vi "stop.vi"(3 "error in (no error)":errorcluster, 4 "stop":bool, 5 "niDAQmxAO in":refnum<class "niDAQmxAO.lvclass">) -> (0 "error out":errorcluster, 1 "Stopped":bool, 2 "niDAQmxAO out":refnum<class "niDAQmxAO.lvclass">)   [LabVIEW 2009, in "Hardware.lvlib" / "Channels.lvlib" / "niDAQmxAO.lvclass"]
uses:
  niDAQmxAO.lvclass
  C:/Program Files/National Instruments/LabVIEW 2009/resource/objmgr/daqmx.rc
panel:
  out "SampQuant.SampPerChan":dbl
  out "TotalSampPerChanGenerated":dbl
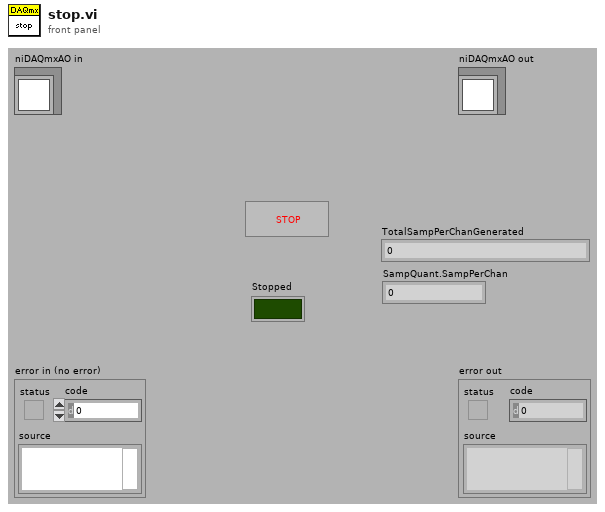
[diagram p1: front panel]
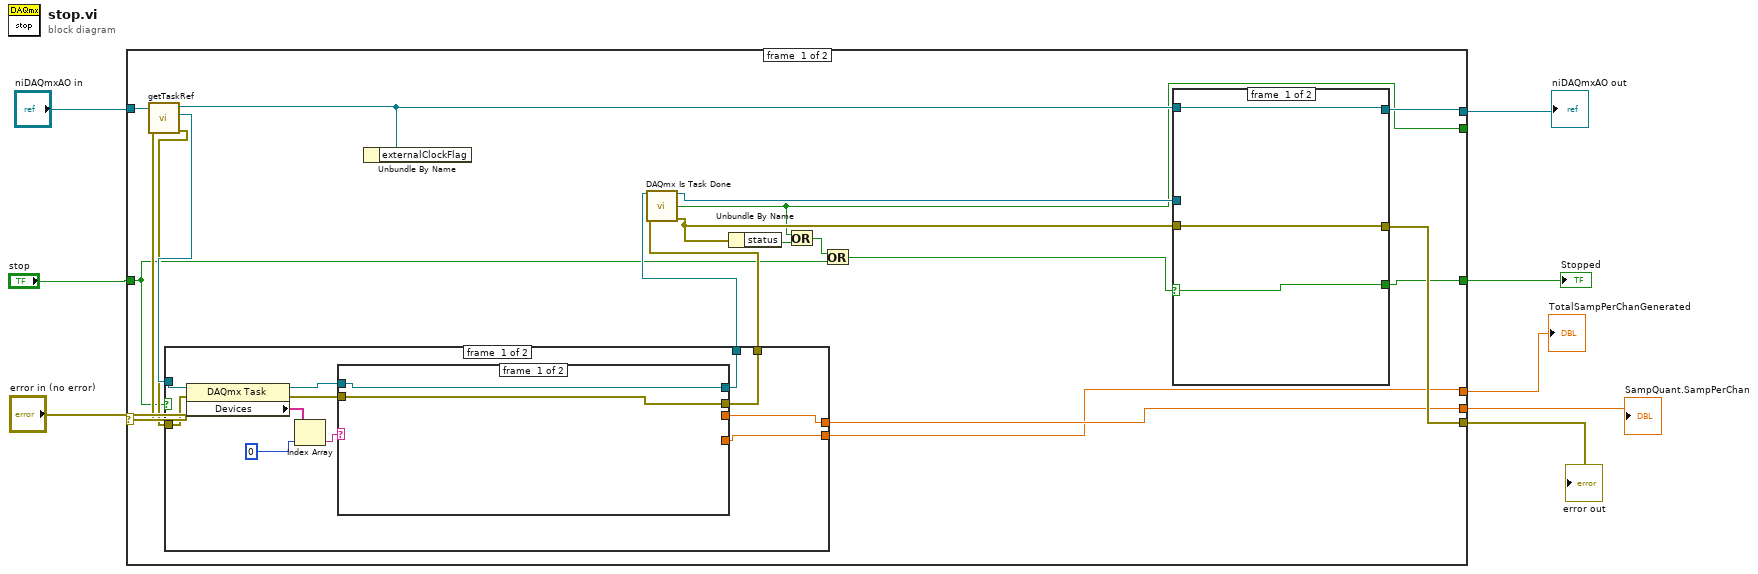
[diagram p0: block diagram]
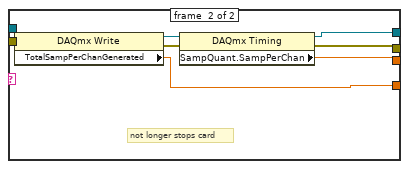
[diagram p2: hidden frame]
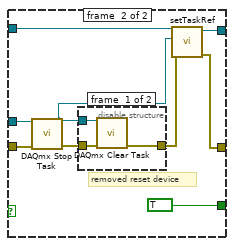
[diagram p4: hidden frame]
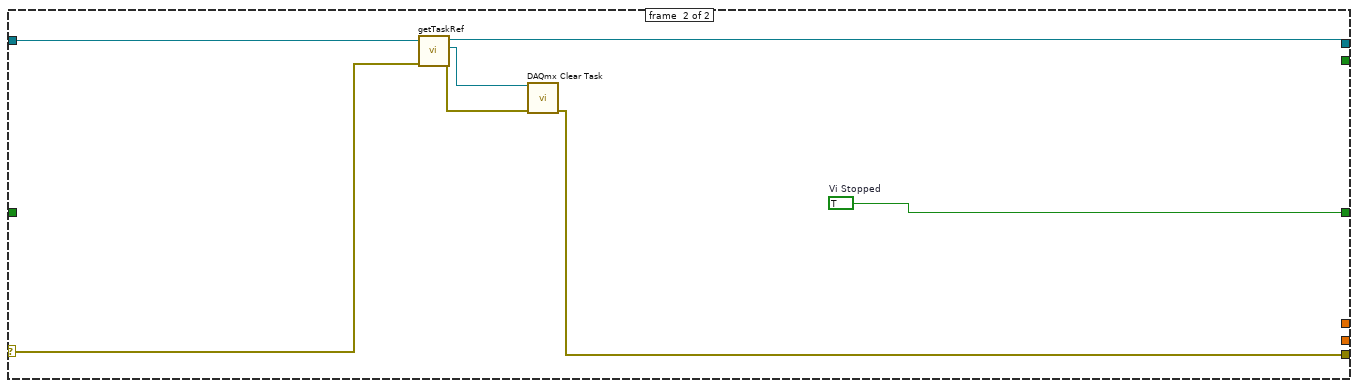
[diagram p6: hidden frame]
diagram:
  n1 = case shown="No Error" "error in (no error)" {
    selector: "error in (no error)" -> [w26 w72]
    tunnel: [w23 w68] -> w7
    tunnel: [w13 w69] -> w5
    tunnel: "niDAQmxAO in" -> [w27 w73]
    tunnel: "stop" -> [w9 _]
    tunnel: [w20 w67] -> w3
    tunnel: [w12 _] -> _
    tunnel: [w15 _] -> w2
    tunnel: [w16 _] -> w1
    frame #0 {
      n2 = call "getTaskRef.vi"("error in (no error)"=w26, "niDAQmxAO.lvclass in"=w27) -> ("error out"=w18:errorcluster, "DAQmx Task Ref"=w19:refnum<k21>, "niDAQmxAO.lvclass out"=w14:refnum<class "niDAQmxAO.lvclass">)  [unwired: 7 in]
      n3 = case shown="False" w9 {
        tunnel: w19 -> [w35 w50]
        tunnel: w18 -> [w34 w49]
        tunnel: [w38 w50] -> w17
        tunnel: [w37 w49] -> w10
        tunnel: [w28 _] -> w16
        tunnel: [w36 _] -> w15
        frame #0 {
          n4 = property class="DAQmx Task"(reference=w35, error in=w34) -> (reference out=w33:refnum<k21>, error out=w32:errorcluster, "Devices"=w30:tag[])
          n5 = Index Array(array=w30, index=0) -> (element=w29:tag)
          n6 = case shown="\"Ao32\", \"Ao8a\", \"DAQ\"" w29 {
            tunnel: [w40 w42] -> w38
            tunnel: [w39 w46] -> w37
            tunnel: [_ w43] -> w36
            tunnel: w33 -> [w40 w45]
            tunnel: w32 -> [w39 w44]
            tunnel: [_ w41] -> w28
            frame #0 {
            }
            frame #1 {
              # "not longer stops card"
              n7 = property class="DAQmx Write"(reference=w45, error in=w44) -> (reference out=w48:refnum<k21>, error out=w47:errorcluster, "TotalSampPerChanGenerated"=w43:dbl)
              n8 = property class="DAQmx Timing"(reference=w48, error in=w47) -> (reference out=w42:refnum<k21>, error out=w46:errorcluster, "SampQuant.SampPerChan"=w41:dbl)
            }
          }
        }
        frame #1 {
        }
      }
      n9 = Unbundle By Name(w14) -> ()  [unwired: 1 out]
      n10 = call <vilib>:"DAQmx Is Task Done.vi"("task/channels in"=w17, "error in"=w10) -> ("task out"=w25:refnum<k21>, "task done?"=w12:bool, "error out"=w24:errorcluster)  [unwired: 11 in]
      n11 = Unbundle By Name(w24) -> ("status"=w21:bool)
      n12 = Or(x=w12, y=w21) -> (x .or. y?=w22:bool)
      n13 = Or(x=w22, y=w9) -> (x .or. y?=w11:bool)
      n14 = case shown="True" w11 {
        selector: w11 -> [w52 _]
        tunnel: w25 -> [_ w60]
        tunnel: w24 -> [w53 w61]
        tunnel: [w53 w58] -> w23
        tunnel: [w52 TRUE] -> w20
        tunnel: w14 -> [w51 w59]
        tunnel: [w51 w57] -> w13
        frame #0 {
        }
        frame #1 {
          # "removed reset device"
          n15 = call <vilib>:"DAQmx Stop Task.vi"("task/channels in"=w60, "error in"=w61) -> ("task out"=w54:refnum<k21>, "error out"=w56:errorcluster)  [unwired: 12 in]
          n16 = disable-structure shown="Enabled" {
            disable-tunnel: w56 -> [w65 w66]
            disable-tunnel: [w64 w66] -> w55
            disable-tunnel: w54 -> [w63 _]
            frame #0 {
              n17 = call <vilib>:"DAQmx Clear Task.vi"("task in"=w63, "error in"=w65) -> ("error out"=w64:errorcluster)  [unwired: 13 in]
            }
            frame #1 {
            }
          }
          n18 = call "setTaskRef.vi"("error in (no error)"=w55, "DAQmx Task Ref"=w54, "niDAQmxAO.lvclass in"=w59) -> ("error out"=w58:errorcluster, "niDAQmxAO.lvclass out"=w57:refnum<class "niDAQmxAO.lvclass">)  [unwired: 7 in]
        }
      }
    }
    frame #1 {
      w67 = TRUE  # Vi Stopped
      n19 = call "getTaskRef.vi"("error in (no error)"=w72, "niDAQmxAO.lvclass in"=w73) -> ("error out"=w70:errorcluster, "DAQmx Task Ref"=w71:refnum<k21>, "niDAQmxAO.lvclass out"=w69:refnum<class "niDAQmxAO.lvclass">)  [unwired: 7 in]
      n20 = call <vilib>:"DAQmx Clear Task.vi"("task in"=w71, "error in"=w70) -> ("error out"=w68:errorcluster)  [unwired: 13 in]
    }
  }
  "error out" <- w7
  "niDAQmxAO out" <- w5
  "Stopped" <- w3
  "TotalSampPerChanGenerated" <- w2
  "SampQuant.SampPerChan" <- w1
